vi "Write Value.vi"(8 "error in (no error)":errorcluster, 10 "Value":dbl, 11 "double in":refnum<class "double.lvclass">) -> (0 "error out":errorcluster, 3 "double out":refnum<class "double.lvclass">)   [LabVIEW 2020, in "Protobuf RAW.lvlib" / "double.lvclass"]
uses:
  double.lvclass
  double.lvclass/double.ctl
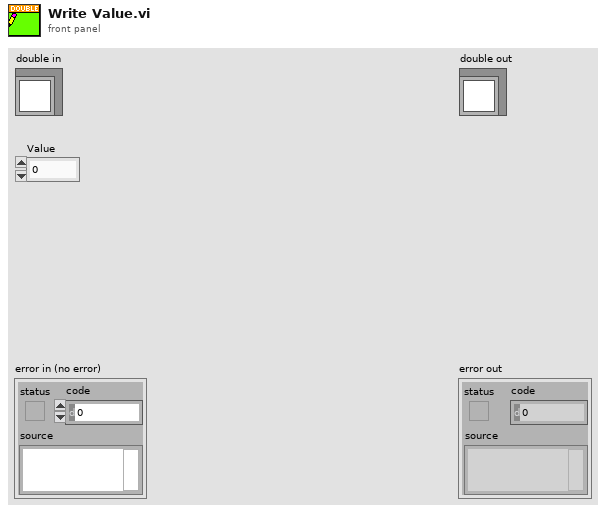
[diagram p1: front panel]
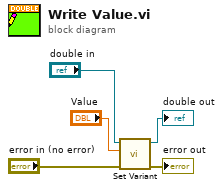
[diagram p0: block diagram]
diagram:
  n1 = call-dynamic "Set Variant.vi"("error in (no error)"="error in (no error)", "Value"="Value", "Proto Type Common in"="double in") -> ("error out"=→"error out":errorcluster, "Proto Type Common out"=→"double out":refnum<class "double.lvclass">)  [unwired: 7 in]
